vi "Grab Weight Precheck.vi"(8 "error in (no error)":errorcluster, 10 "Weight Number":i32, 11 "GrabberTool Class in":refnum<class "GrabberTool Class.lvclass">) -> (0 "error out":errorcluster, 3 "GrabberTool Class out":refnum<class "GrabberTool Class.lvclass">)   [LabVIEW 2017, in "GrabberTool Class.lvclass"]
uses:
  GrabberTool Class.lvclass
  WorkTable Class/WorkTable Class.lvclass
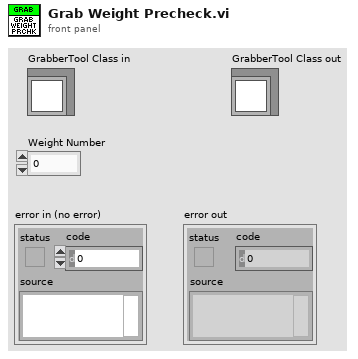
[diagram p1: front panel]
types:
  T1 = typedef "Worktable_Weights.ctl" = cluster{"Weight Slots":T2[], "Vacuum Channel":i32}
  T2 = typedef "Worktable_Weight.ctl" = cluster{"Weight State":enum16{"Empty", "Populated"}, "Weight Type":T3, "Location/Orientation":T4}
  T3 = typedef "Weight Type.ctl" = enum16{"Weight 1", "Weight 2", "Weight 3", "Weight 4", "Weight 5", "Weight 6", "Weight 7", "Weight 8", "Weight 9", "Weight 10", "Weight 11", "Weight 12", "Weight 13", "Weight 14", "Weight 15", "Weight 16"}
  T4 = typedef "Position_Orientation.ctl" = cluster{"Center":refnum<class "Vec3d Class.lvclass">, "Orientation":refnum<class "Orient3d Class.lvclass">}
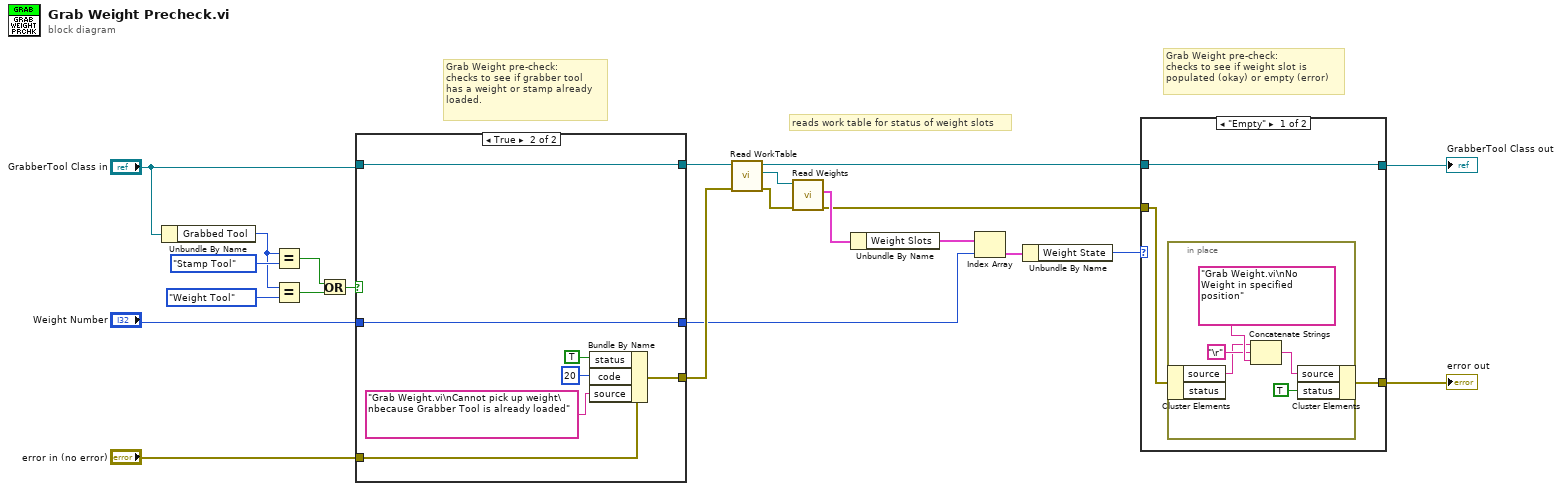
[diagram p0: block diagram]
diagram:
  # "Grab Weight pre-check:\nchecks to see if weight slot is\npopulated (okay) or empty (error)"
  # "reads work table for status of weight slots"
  # "Grab Weight pre-check:\nchecks to see if grabber tool\nhas a weight or stamp already \nloaded."
  n1 = Unbundle By Name("GrabberTool Class in") -> ("Grabbed Tool"=w18:enum16{"Weight Tool", "Stamp Tool", "Nothing"})
  n2 = Equal?(x=w18, y=enum16{"Weight Tool", "Stamp Tool", "Nothing"}."Stamp Tool") -> (x = y?=w20:bool)
  n3 = Equal?(x=w18, y=enum16{"Weight Tool", "Stamp Tool", "Nothing"}."Weight Tool") -> (x = y?=w19:bool)
  n4 = Or(x=w20, y=w19) -> (x .or. y?=w21:bool)
  n5 = case shown="True" w21 {
    tunnel: [w25 w32] -> w13
    tunnel: "GrabberTool Class in" -> [w25 w32]
    tunnel: [w24 w30] -> w12
    tunnel: "error in (no error)" -> [w24 w31]
    tunnel: [w23 w26] -> w7
    tunnel: "Weight Number" -> [w23 w26]
    frame False {
    }
    frame True {
      n6 = Bundle By Name(cluster=w31, "status"=TRUE, "code"=20, "source"="Grab Weight.vi\nCannot pick up weight\nbecause Grabber Tool is already loaded") -> (w30:errorcluster)
    }
  }
  n7 = call-dynamic "Read WorkTable.vi"("error in"=w12, "Gantry Class in"=w13) -> ("error out"=w10:errorcluster, "Worktable"=w11:refnum<class "FlexWorktable.lvclass">, "Gantry Class out"=w4:refnum<class "GrabberTool Class.lvclass">)  [unwired: 7 in]
  n8 = call-dynamic "Read Weights.vi"("error in (no error)"=w10, "WorkTable Class in"=w11) -> ("error out"=w2:errorcluster, "Weights"=w9:T1)  [unwired: 7 in, 1 out]
  n9 = Unbundle By Name(w9) -> ("Weight Slots"=w8:T2[])
  n10 = Index Array(array=w8, index=w7) -> (element=w6:T2)
  n11 = Unbundle By Name(w6) -> ("Weight State"=w5:enum16{"Empty", "Populated"})
  n12 = case shown="\"Empty\"" w5 {
    tunnel: w4 -> [w35 w42]
    tunnel: [w35 w42] -> w3
    tunnel: w2 -> [w34 w41]
    tunnel: [w33 w41] -> w1
    frame "Empty" {
      n13 = in-place {
        n14 = in-place-cluster #1(w34) -> ("source"=w37:string)  [unwired: 1 out]
        n15 = Concatenate Strings(w37, "\r", "Grab Weight.vi\nNo Weight in specified position" ("string")) -> (w38:string)
        n16 = in-place-cluster #1("source"=w38, "status"=TRUE) -> (w33:errorcluster)
      }
    }
    frame "Populated" {
    }
  }
  "error out" <- w1
  "GrabberTool Class out" <- w3
